vi "Shared Variable Management Loop.vi"(8 "error in (no error)":errorcluster, 11 "Message Queues":T1) -> (0 "error out":errorcluster)   [LabVIEW 2024]
doc: "Creates server processes in the shared variable engine and creates, updates, and destroys the I/O points in the server processes. This is a working thread of the server and is responsible for shared variables management."
uses:
  Shared/Message Queue/Server Message Queues.ctl
  Shared/Message Queue/Message Cluster.ctl
  Globals/Global - Server.vi
  Shared/Message Queue.lvlib
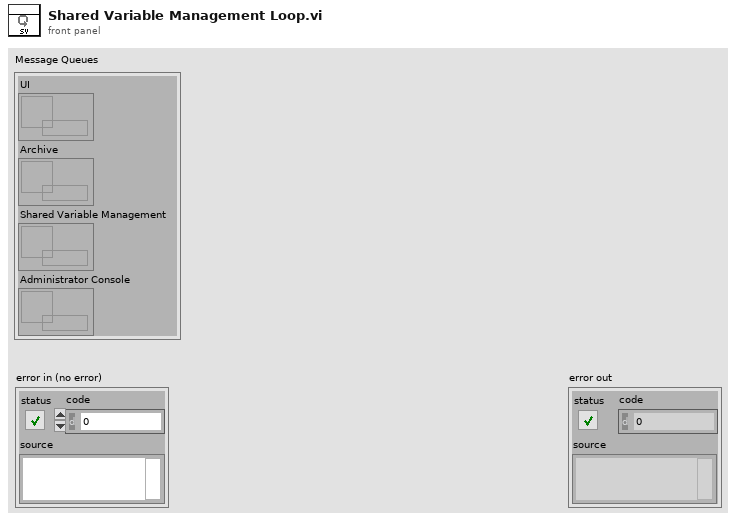
[diagram p1: front panel]
types:
  T1 = typedef "Message Queue.lvlib/Server Message Queues.ctl" = cluster{"UI":refnum<queue>, "Archive":refnum<queue>, "Shared Variable Management":refnum<queue>, "Administrator Console":refnum<queue>}
  T2 = typedef "Subsystem IO Attributes.ctl" = cluster{"Name":string, "Data Type":enum32{"u32BitField", "bool", "double", "string", "int8", "uint8", "int16", "uint16", "int32", "uint32", "int64", "uint64", "single", "double waveform", "int16 waveform", "array of boolean", "array of int8", "array of uint8", "array of int16", "array of uint16", "array of int32", "array of uint32", "array of int64", "array of uint64", "array of single", "array of double", "array of double waveform", "array of int16 waveform", "array of string", "variant", "timestamp", "fixed point", "custom"}, "Access Type":enum32{"Read only", "Write only", "Read/write"}, "Alarm Enabled?":bool, "Logging Enabled?":bool, "Logging Attributes":T3, "Alarm Attributes":T4}
  T3 = typedef "Subsystem IO Logging Attributes.ctl" = cluster{"log data? (F)":bool, "log alarms & events? (F)":bool}
  T4 = typedef "Subsystem IO Alarm Attributes.ctl" = cluster{"Hi:enable? (F)":bool, "Hi:name":string, "Hi:level/change":dbl, "Lo:enable? (F)":bool, "Lo:name":string, "Lo:level/change":dbl, "Boolean:enable? (F)":bool, "Boolean:name":string, "Boolean:value":bool, "BadStatus:enable? (F)":bool, "BadStatus:name":string}
  T5 = typedef "System Configuration.ctl" = cluster{"Name":string, "Description":string, "Logging Computer Name":string, "Logging Database Name":string, "Logging Database Path":path, "Archive Computer Name":string, "Archive Database Name":string, "Archive Database Path":path, "Lifespan (days)":u32, "Archive Enabled":bool, "Archive Interval (hours)":u32, "Subsystems":T6[]}
  T6 = typedef "Subsystem Configuration.ctl" = cluster{"Name":string, "Root URL":refnum<k21>}
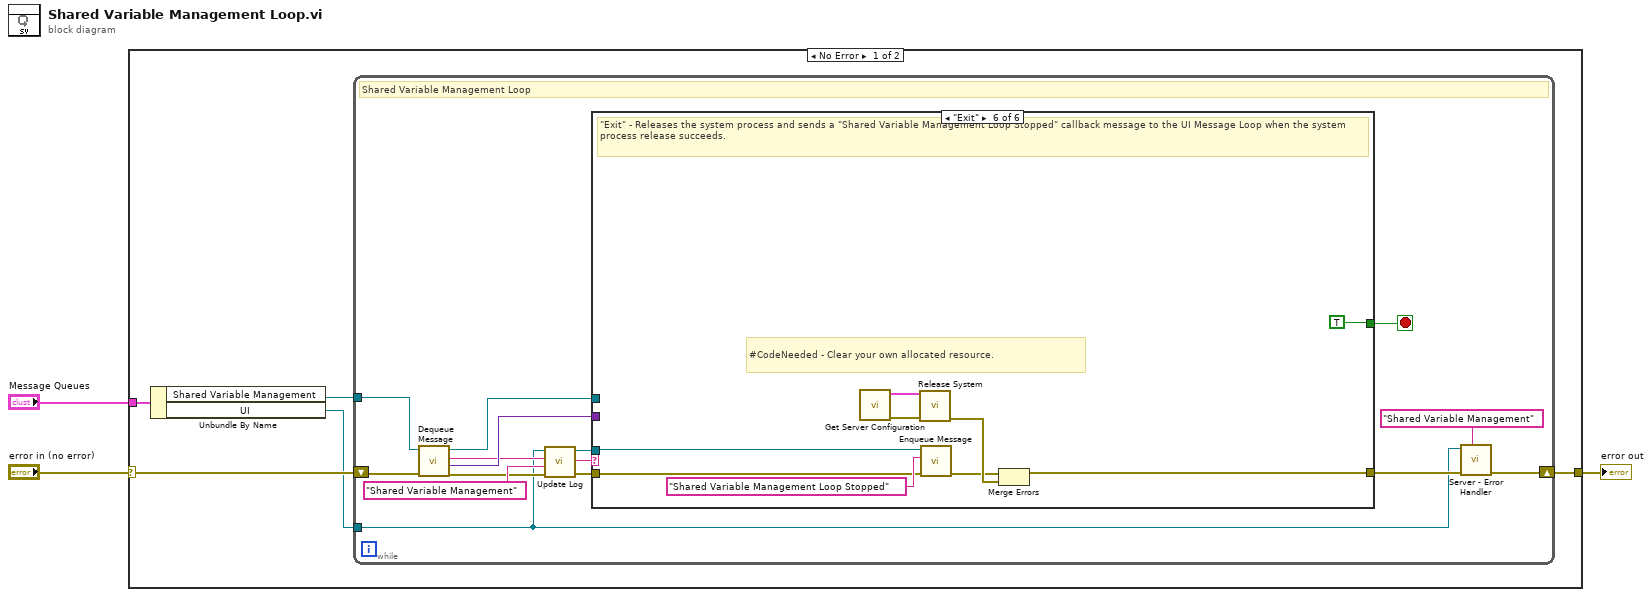
[diagram p0: block diagram]
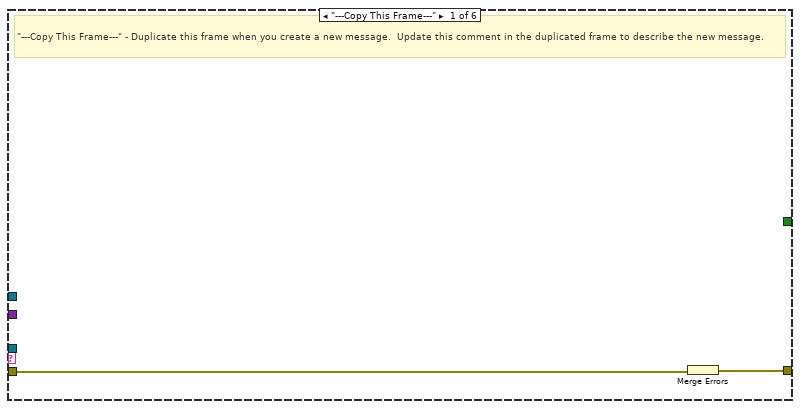
[diagram p2: hidden frame]
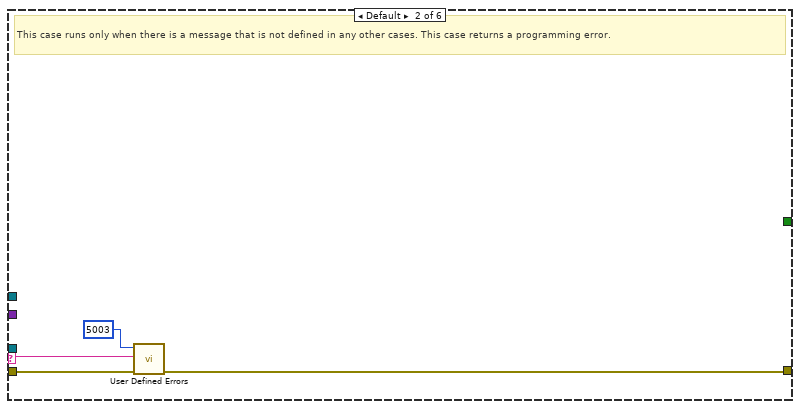
[diagram p3: hidden frame]
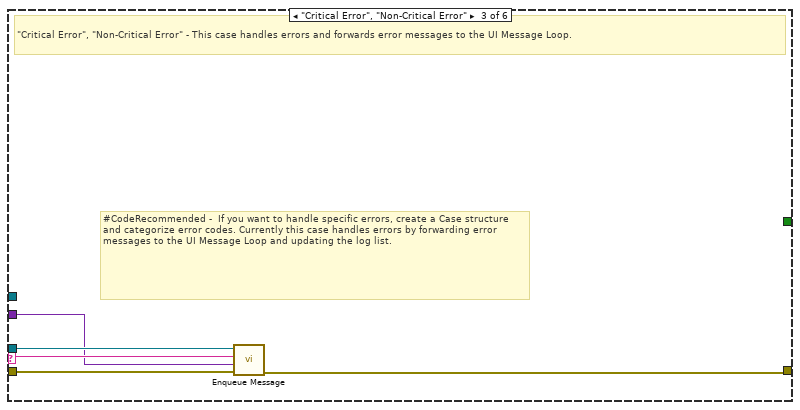
[diagram p4: hidden frame]
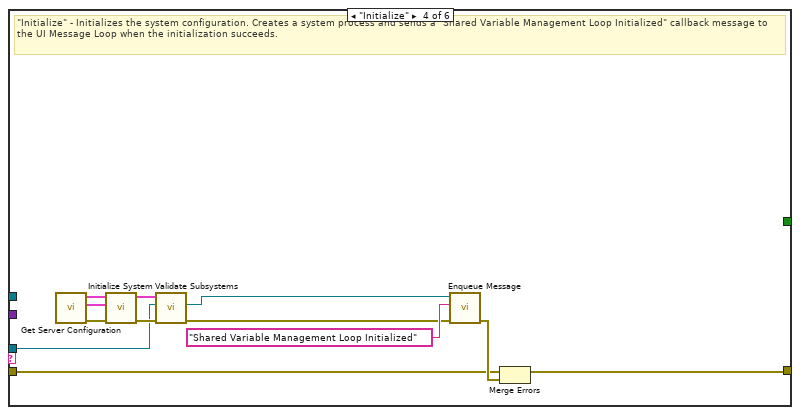
[diagram p5: hidden frame]
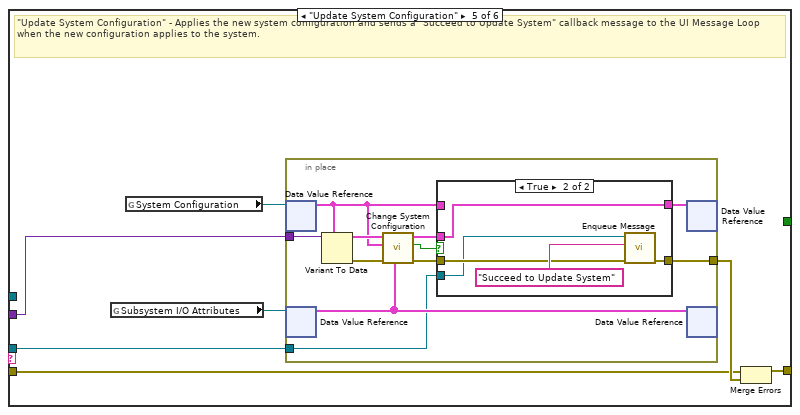
[diagram p6: hidden frame]
diagram:
  n1 = case shown="No Error" "error in (no error)" {
    selector: "error in (no error)" -> [w5 w81]
    tunnel: "Message Queues" -> [w8 _]
    tunnel: [w6 w81] -> w1
    frame No Error {
      n2 = Unbundle By Name(w8) -> ("Shared Variable Management"=w7:refnum<queue>, "UI"=w4:refnum<queue>)
      n3 = while {
        tunnel: w7 -> [w12]
        shift-right: [w13] -> w6
        shift-left: w5 -> [w22]
        tunnel: w4 -> [w11]
        stop <- w23 stop-if-true
        # "Shared Variable Management Loop"
        n4 = call "Dequeue Message.vi"("error in (no error)"=w22, "Message Queue"=w12) -> ("error out"=w15:errorcluster, "Message Data"=w21:variant, "Message"=w18:string, "dup Message Queue"=w20:refnum<queue>)  [unwired: 6 in]
        n5 = call "Update Log.vi"("error in (no error)"=w15, "Component"="Shared Variable Management", "Status"=w18, "UI Message Queue"=w11) -> ("error out"=w16:errorcluster, "dup Status"=w17:string, "dup UI Message Queue"=w10:refnum<queue>)  [unwired: 5 in]
        n6 = case "Message Cases" shown="\"Exit\"" w17 {
          selector: w17 -> [_ w27 w33 _ _ _]
          tunnel: w20 -> [_ _ _ _ _ _]
          tunnel: [w25 w28 w30 w45 w50 w78] -> w14
          tunnel: [_ _ _ _ _ TRUE] -> w23
          tunnel: w21 -> [_ _ w32 _ w51 _]
          tunnel: w16 -> [w24 w26 w31 w42 w47 w76]
          tunnel: w10 -> [_ _ w34 w35 w49 w77]
          frame "---Copy This Frame---" {
            # "\"---Copy This Frame---\" - Duplicate this frame when you create a new message.  Update this comment in the duplicated frame to describe the new message."
            n7 = Merge Errors(w24) -> (w25:errorcluster)
          }
          frame Default {
            # "This case runs only when there is a message that is not defined in any other cases. This case returns a programming error."
            n8 = call "User Defined Errors.vi"("error in (no error)"=w26, "Parameter 1"=w27, "Error Code (0)"=5003 ("error code (0)")) -> ("error out"=w28:errorcluster)  [unwired: 8 in]
          }
          frame "Critical Error", "Non-Critical Error" {
            # "#CodeRecommended -  If you want to handle specific errors, create a Case structure and categorize error codes. Currently this case handles errors by forwarding error messages to the UI Message Loop and updating the log list."
            # "\"Critical Error\", \"Non-Critical Error\" - This case handles errors and forwards error messages to the UI Message Loop."
            n9 = call "Enqueue Message.vi"("error in (no error)"=w31, "Message Data"=w32, "Message"=w33, "Message Queue"=w34) -> ("error out"=w30:errorcluster)  [unwired: 6 in, 1 out]
          }
          frame "Initialize" {
            # "\"Initialize\" - Initializes the system configuration. Creates a system process and sends a \"Shared Variable Management Loop Initialized\" callback message to the UI Message Loop when the initialization succeeds."
            n10 = call "Get Server Configuration.vi"() -> ("error out"=w41:errorcluster, "Subsystem I/O Attributes"=w43:T2[], "System Configuration"=w40:T5)  [unwired: 9 in]
            n11 = call "Initialize System.vi"("error in (no error)"=w41, "Subsystem I/O Attributes"=w43, "System Configuration In"=w40) -> ("error out"=w39:errorcluster, "System Configuration Out"=w37:T5)  [unwired: 7 in]
            n12 = call "Validate Subsystems.vi"("error in (no error)"=w39, "UI Message Queue In"=w35, "System Configuration"=w37) -> ("error out"=w38:errorcluster, "UI Message Queue Out"=w36:refnum<queue>)  [unwired: 6 in, 1 out]
            n13 = call "Enqueue Message.vi"("error in (no error)"=w38, "Message"="Shared Variable Management Loop Initialized", "Message Queue"=w36) -> ("error out"=w44:errorcluster)  [unwired: 7 in, 1 out]
            n14 = Merge Errors(w42, w44) -> (w45:errorcluster)
          }
          frame "Update System Configuration" {
            # "\"Update System Configuration\" - Applies the new system configuration and sends a \"Succeed to Update System\" callback message to the UI Message Loop when the new configuration applies to the system."
            n15 = global read "Global - Server.vi" "Subsystem I/O Attributes"() -> (w53:refnum<data-value>)
            n16 = global read "Global - Server.vi" "System Configuration"() -> (w52:refnum<data-value>)
            n17 = in-place {
              in-place-border: [w60] -> w48
              in-place-border: w51 -> [w55]
              in-place-border: w49 -> [w54]
              n18 = in-place-dvr #1(w52) -> (w56:T5)  [unwired: 1 out]
              n19 = in-place-dvr #2(w53) -> (w64:T2[])  [unwired: 1 out]
              n20 = Variant To Data(type=w56, Variant=w55) -> (data=w58:T5, error out=w57:errorcluster)  [unwired: 1 in]
              n21 = call "Change System Configuration.vi"("Subsystem I/O Attributes"=w64, "error in (no error)"=w57, "Old System Configuration"=w56, "System Configuration"=w58) -> ("error out"=w62:errorcluster, "Succeed?"=w63:bool, "dup System Configuration"=w61:T5)  [unwired: 5 in]
              n22 = case shown="True" w63 {
                tunnel: w62 -> [w66 w70]
                tunnel: w61 -> [_ w68]
                tunnel: w56 -> [w65 _]
                tunnel: [w66 w69] -> w60
                tunnel: [w65 w68] -> w59
                tunnel: w54 -> [_ w67]
                frame False {
                }
                frame True {
                  n23 = call "Enqueue Message.vi"("error in (no error)"=w70, "Message"="Succeed to Update System", "Message Queue"=w67) -> ("error out"=w69:errorcluster)  [unwired: 7 in, 1 out]
                }
              }
              n24 = in-place-dvr #1(w59) -> ()  [unwired: 2 out]
              n25 = in-place-dvr #2(w64) -> ()  [unwired: 2 out]
            }
            n26 = Merge Errors(w47, w48) -> (w50:errorcluster)
          }
          frame "Exit" {
            # "#CodeNeeded - Clear your own allocated resource."
            # "\"Exit\" - Releases the system process and sends a \"Shared Variable Management Loop Stopped\" callback message to the UI Message Loop when the system process release succeeds."
            n27 = call "Get Server Configuration.vi"() -> ("error out"=w73:errorcluster, "System Configuration"=w74:T5)  [unwired: 9 in, 1 out]
            n28 = call "Release System.vi"("error in (no error)"=w73, "System Configuration"=w74) -> ("error out"=w75:errorcluster)  [unwired: 9 in]
            n29 = call "Enqueue Message.vi"("error in (no error)"=w76, "Message"="Shared Variable Management Loop Stopped", "Message Queue"=w77) -> ("error out"=w72:errorcluster)  [unwired: 7 in, 1 out]
            n30 = Merge Errors(w72, w75) -> (w78:errorcluster)
          }
        }
        n31 = call "Server - Error Handler.vi"("Component"="Shared Variable Management", "error in (no error)"=w14, "Message Queue"=w11) -> ("error out"=w13:errorcluster)  [unwired: 8 in]
      }
    }
    frame Error {
    }
  }
  "error out" <- w1
